vi "Run.vi"(8 "error in (no error)":errorcluster, 11 "BaseDriver in":refnum<class "BaseDriver.lvclass">) -> (0 "error out":errorcluster, 3 "BaseDriver out":refnum<class "BaseDriver.lvclass">)   [LabVIEW 2013, in "BaseDriver.lvclass"]
doc: "This is the main loop of the driver.\nAfter setting up your driver, call this VI to actually run it."
uses:
  BaseDriver.lvclass
  BaseDriver.lvclass/BaseDriver.ctl
  Reader/BaseReader/BaseReader.lvclass
  Message/BaseMessage/BaseMessage.lvclass
  Responder/BaseResponder/BaseResponder.lvclass
  global_stop.vi
  Read Reconnect.vi
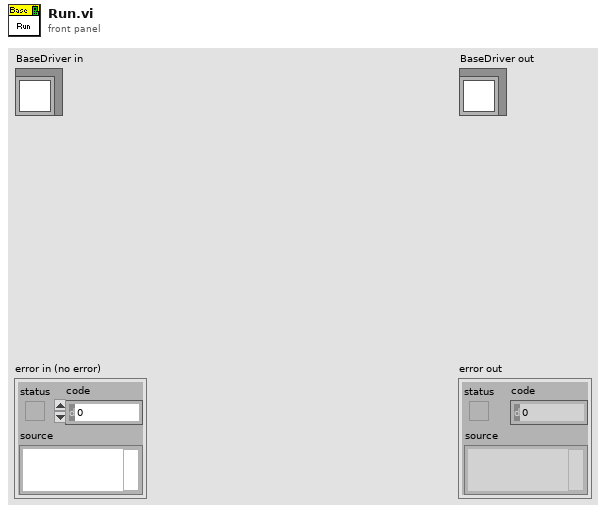
[diagram p1: front panel]
types:
  T1 = typedef "message_queue.ctl" = refnum<queue>
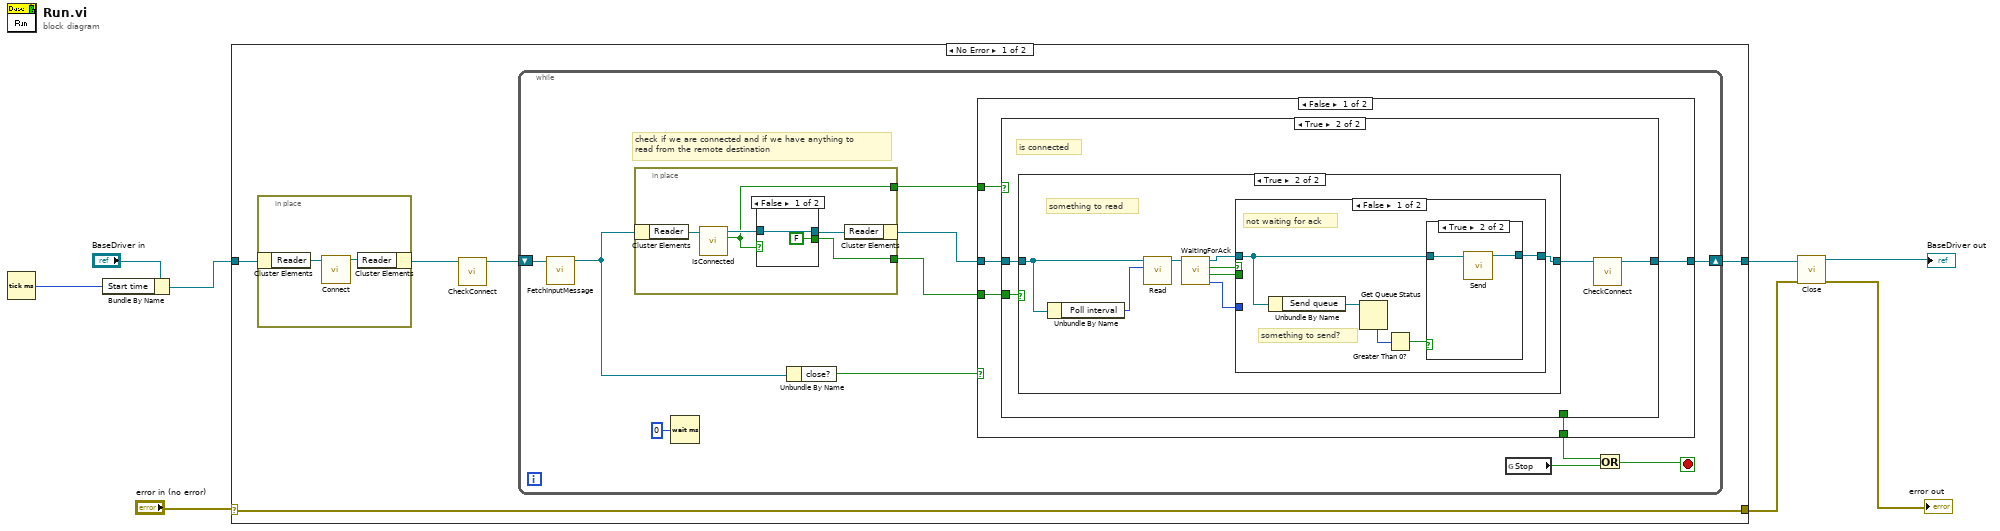
[diagram p0: block diagram]
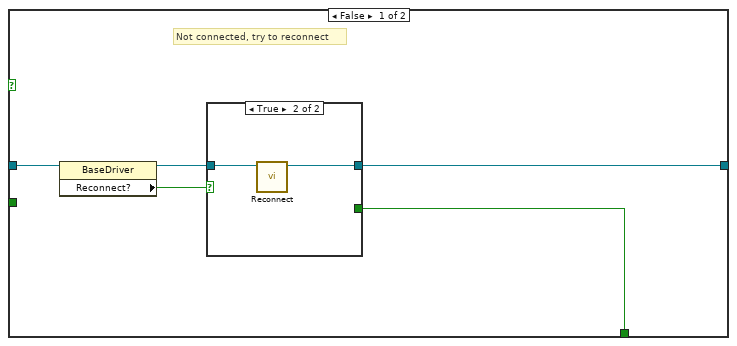
[diagram p2: hidden frame]
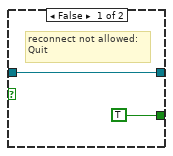
[diagram p3: hidden frame]
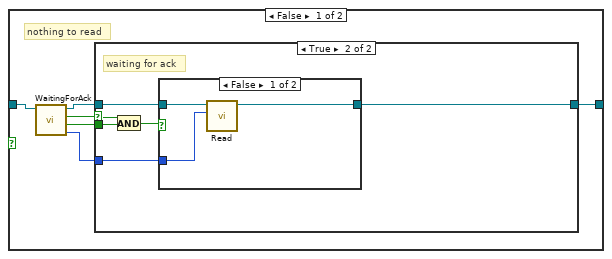
[diagram p4: hidden frame]
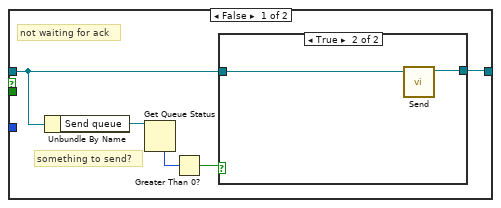
[diagram p5: hidden frame]
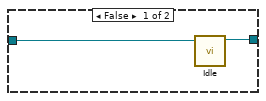
[diagram p6: hidden frame]
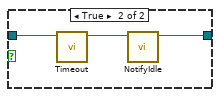
[diagram p7: hidden frame]
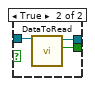
[diagram p11: hidden frame]
diagram:
  n1 = Tick Count (ms)() -> (millisecond timer value=w2:u32)
  n2 = Bundle By Name(cluster="BaseDriver in", "Start time"=w2) -> (w1:refnum<class "BaseDriver.lvclass">)
  n3 = case shown="No Error" "error in (no error)" {
    selector: "error in (no error)" -> [w12 w101]
    tunnel: w1 -> [w11 w102]
    tunnel: [w13 w102] -> w7
    tunnel: [w12 w101] -> w5
    frame No Error {
      n4 = in-place {
        n5 = in-place-cluster #1(w11) -> ("Reader"=w15:refnum<class "BaseReader.lvclass">)
        n6 = call-dynamic "Connect.vi"("BaseReader in"=w15) -> ("BaseReader out"=w14:refnum<class "BaseReader.lvclass">)  [unwired: 9 in, 1 out]
        n7 = in-place-cluster #1("Reader"=w14) -> (w10:refnum<class "BaseDriver.lvclass">)
      }
      n8 = call "CheckConnect.vi"("BaseDriver in"=w10) -> ("BaseDriver out"=w9:refnum<class "BaseDriver.lvclass">)  [unwired: 9 in, 1 out]
      n9 = while {
        shift-right: [w26] -> w13
        shift-left: w9 -> [w23]
        stop <- w19 stop-if-true
        # "check if we are connected and if we have anything to\nread from the remote destination"
        n10 = call "FetchInputMessage.vi"("BaseDriver in"=w23) -> ("BaseDriver out"=w22:refnum<class "BaseDriver.lvclass">)  [unwired: 9 in, 1 out]
        n11 = in-place {
          in-place-border: [w95] -> w17
          in-place-border: [w91] -> w24
          n12 = in-place-cluster #2(w22) -> ("Reader"=w93:refnum<class "BaseReader.lvclass">)
          n13 = call-dynamic "IsConnected.vi"("BaseReader in"=w93) -> ("connected?"=w91:bool, "BaseReader out"=w92:refnum<class "BaseReader.lvclass">)  [unwired: 8 in, 1 out]
          n14 = case shown="False" w91 {
            tunnel: [FALSE ("Data available?") w100] -> w95
            tunnel: [w97 w99] -> w94
            tunnel: w92 -> [w97 w98]
            frame False {
            }
            frame True {
              n15 = call-dynamic "DataToRead.vi"("BaseReader in"=w98) -> ("Data available?"=w100:bool, "BaseReader out"=w99:refnum<class "BaseReader.lvclass">)  [unwired: 8 in, 1 out]
            }
          }
          n16 = in-place-cluster #2("Reader"=w94) -> (w25:refnum<class "BaseDriver.lvclass">)
        }
        n17 = Wait (ms)(milliseconds to wait=u32 0) -> ()  [unwired: 1 out]
        n18 = Unbundle By Name(w22) -> ("close?"=w21:bool)
        n19 = case shown="False" w21 {
          selector: w21 -> [_ w90]
          tunnel: w17 -> [w31 _]
          tunnel: [w30 w89] -> w26
          tunnel: w25 -> [w29 w89]
          tunnel: w24 -> [w28 _]
          tunnel: [w27 w90] -> w18
          frame False {
            n20 = case shown="True" w28 {
              tunnel: w31 -> [_ w44]
              tunnel: [w36 w41] -> w30
              tunnel: w29 -> [w35 w43]
              tunnel: [w32 _] -> w27
              frame False {
                # "Not connected, try to reconnect"
                n21 = property class="BaseDriver"(reference=w35) -> (reference out=w34:refnum<class "BaseDriver.lvclass">, "Reconnect?"=w33:bool)  [unwired: 1 in, 1 out]
                n22 = case shown="True" w33 {
                  tunnel: [w38 w39] -> w36
                  tunnel: w34 -> [w38 w40]
                  tunnel: [TRUE _] -> w32
                  frame False {
                    # "reconnect not allowed:\nQuit"
                  }
                  frame True {
                    n23 = call "Reconnect.vi"("BaseDriver in"=w40) -> ("BaseDriver out"=w39:refnum<class "BaseDriver.lvclass">)  [unwired: 9 in, 1 out]
                  }
                }
              }
              frame True {
                # "is connected"
                n24 = case shown="True" w44 {
                  tunnel: w43 -> [w50 w79]
                  tunnel: [w46 w72] -> w42
                  frame False {
                    # "nothing to read"
                    n25 = call "WaitingForAck.vi"("BaseDriver in"=w50) -> ("Time left"=w45:u32, "Timed out?"=w48:bool, "Waiting?"=w49:bool, "BaseDriver out"=w47:refnum<class "BaseDriver.lvclass">)  [unwired: 7 in]
                    n26 = case shown="True" w49 {
                      selector: w49 -> [_ w65]
                      tunnel: w48 -> [_ w64]
                      tunnel: w47 -> [w52 w63]
                      tunnel: [w51 w62] -> w46
                      tunnel: w45 -> [_ w60]
                      frame False {
                        # "something to send?"
                        # "not waiting for ack"
                        n27 = Unbundle By Name(w52) -> ("Send queue"=w55:T1)
                        n28 = Get Queue Status(queue=w55) -> (# elements in queue=w54:i32)  [unwired: 2 in, 7 out]
                        n29 = Greater Than 0?(x=w54) -> (x > 0?=w53:bool)
                        n30 = case shown="True" w53 {
                          tunnel: w52 -> [w57 w59]
                          tunnel: [w56 w58] -> w51
                          frame False {
                            n31 = call "Idle.vi"("BaseDriver in"=w57) -> ("BaseDriver out"=w56:refnum<class "BaseDriver.lvclass">)  [unwired: 9 in, 1 out]
                          }
                          frame True {
                            n32 = call "Send.vi"("BaseDriver in"=w59) -> ("BaseDriver out"=w58:refnum<class "BaseDriver.lvclass">)  [unwired: 9 in, 1 out]
                          }
                        }
                      }
                      frame True {
                        # "waiting for ack"
                        n33 = And(x=w65, y=w64) -> (x .and. y?=w61:bool)
                        n34 = case shown="False" w61 {
                          tunnel: w63 -> [w68 w71]
                          tunnel: [w67 w69] -> w62
                          tunnel: w60 -> [w66 _]
                          frame False {
                            n35 = call "Read.vi"("Timeout"=w66, "BaseDriver in"=w68) -> ("BaseDriver out"=w67:refnum<class "BaseDriver.lvclass">)  [unwired: 8 in, 1 out]
                          }
                          frame True {
                            n36 = call-dynamic "Timeout.vi"("BaseDriver in"=w71) -> ("BaseDriver out"=w70:refnum<class "BaseDriver.lvclass">)  [unwired: 8 in, 2 out]
                            n37 = call "NotifyIdle.vi"("BaseDriver in"=w70) -> ("BaseDriver out"=w69:refnum<class "BaseDriver.lvclass">)  [unwired: 9 in, 1 out]
                          }
                        }
                      }
                    }
                  }
                  frame True {
                    # "something to read"
                    n38 = Unbundle By Name(w79) -> ("Poll interval"=w78:i32)
                    n39 = call "Read.vi"("Timeout"=w78, "BaseDriver in"=w79) -> ("BaseDriver out"=w73:refnum<class "BaseDriver.lvclass">)  [unwired: 8 in, 1 out]
                    n40 = call "WaitingForAck.vi"("BaseDriver in"=w73) -> ("Time left"=w74:u32, "Timed out?"=w76:bool, "Waiting?"=w77:bool, "BaseDriver out"=w75:refnum<class "BaseDriver.lvclass">)  [unwired: 7 in]
                    n41 = case shown="False" w77 {
                      tunnel: w76 -> [_ _]
                      tunnel: w75 -> [w81 w88]
                      tunnel: [w80 w88] -> w72
                      tunnel: w74 -> [_ _]
                      frame False {
                        # "something to send?"
                        # "not waiting for ack"
                        n42 = Unbundle By Name(w81) -> ("Send queue"=w84:T1)
                        n43 = Get Queue Status(queue=w84) -> (# elements in queue=w83:i32)  [unwired: 2 in, 7 out]
                        n44 = Greater Than 0?(x=w83) -> (x > 0?=w82:bool)
                        n45 = case shown="True" w82 {
                          tunnel: w81 -> [w85 w87]
                          tunnel: [w85 w86] -> w80
                          frame False {
                          }
                          frame True {
                            n46 = call "Send.vi"("BaseDriver in"=w87) -> ("BaseDriver out"=w86:refnum<class "BaseDriver.lvclass">)  [unwired: 9 in, 1 out]
                          }
                        }
                      }
                      frame True {
                      }
                    }
                  }
                }
                n47 = call "CheckConnect.vi"("BaseDriver in"=w42) -> ("BaseDriver out"=w41:refnum<class "BaseDriver.lvclass">)  [unwired: 9 in, 1 out]
              }
            }
          }
          frame True {
          }
        }
        n48 = global read "global_stop.vi" "Stop"() -> (w20:bool)
        n49 = Or(x=w18, y=w20) -> (x .or. y?=w19:bool)
      }
    }
    frame Error {
    }
  }
  n50 = call-dynamic "Close.vi"("error in (no error)"=w5, "BaseDriver in"=w7) -> ("error out"=→"error out":errorcluster, "BaseDriver out"=→"BaseDriver out":refnum<class "BaseDriver.lvclass">)  [unwired: 8 in]
